vi "Update Configured Steps.vi"(6 "Parameters In":variant, 9 "Step Number":i32, 10 "Step Name":string, 11 "Configured Steps In":T1[](array[typedef])) -> (3 "Configured Steps Out":T1[](array[typedef]))   [LabVIEW 2018]
doc: "This VI updates the Configured Steps array. If the control step has not previously been added to the array, it is added to the array, along with its associated configuration parameters. For a pre-existing step, the configuration parameters are updated in the array."
uses:
  controls/Configured Step.ctl
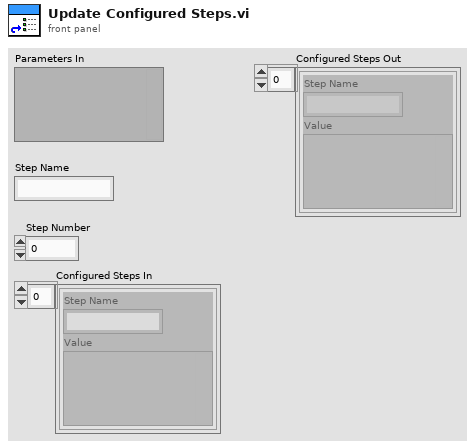
[diagram p1: front panel]
types:
  T1 = typedef "Configured Step.ctl" = cluster{"Step Name":string, "Value":variant}
  T2 = cluster{"Step Name":string, "Parameters In":variant}
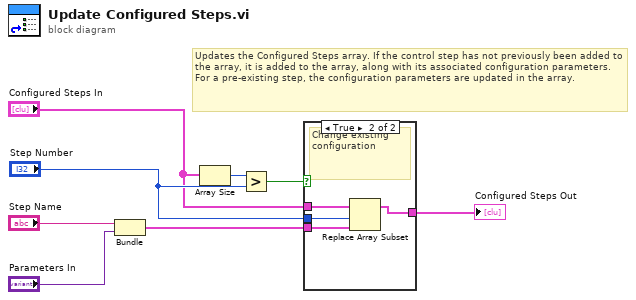
[diagram p0: block diagram]
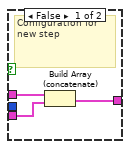
[diagram p2: hidden frame]
diagram:
  # "Updates the Configured Steps array. If the control step has not previously been added to the array, it is added to the array, along with its associated configuration parameters. For a pre-existing step, the configuration parameters are updated in the array."
  n1 = Bundle("Step Name"="Step Name", "Parameters In"="Parameters In") -> (w2:T2)  [unwired: 1 in]
  n2 = Array Size(array="Configured Steps In") -> (size(s)=w5:i32)
  n3 = Greater?(x=w5, y="Step Number") -> (0:w6:bool)
  n4 = case shown="True" w6 {
    tunnel: w2 -> [w9 w12]
    tunnel: [w11 w13] -> w3
    tunnel: "Configured Steps In" -> [w10 w15]
    tunnel: "Step Number" -> [_ w14]
    frame False {
      # "Configuration for\nnew step"
      n5 = Build Array (concatenate)(w10, w9) -> (w11:T1[])
    }
    frame True {
      # "Change existing\nconfiguration"
      n6 = Replace Array Subset(array=w15, new element=w12, index=w14) -> (w13:T1[])
    }
  }
  "Configured Steps Out" <- w3
